vi "Set Handle on Open.vi"(0 "error in":errorcluster, 1 "All Handles ref":refnum<vi>, 2 "hDevice":i32, 3 "Selected Device":i32, 4 "Ch refs":refnum<vi>[](array[refnum]), 5 "OphirLMMeasurementLib.ICoLMMeasurement":refnum<k7>, 8 "Devices List box ref":refnum<vi>) -> ()   [LabVIEW 2017, in "Powermeter_library.lvlib"]
uses:
  Powermeter_library.lvlib
  Channel States.ctl
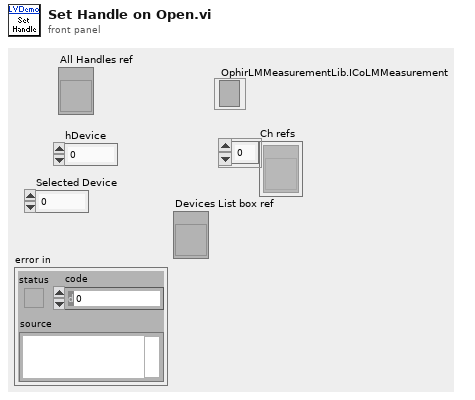
[diagram p1: front panel]
types:
  T1 = typedef "Powermeter_library.lvlib/Channel States.ctl" = enum16{"Init", "Poll", "Set Handle", "Measure"}
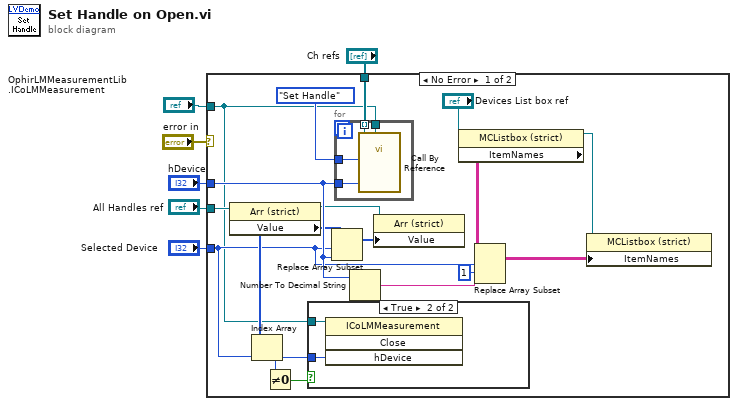
[diagram p0: block diagram]
diagram:
  n1 = case shown="No Error" "error in" {
    tunnel: "Selected Device" -> [w10 _]
    tunnel: "hDevice" -> [w19 _]
    tunnel: "Ch refs" -> [w21 _]
    tunnel: "OphirLMMeasurementLib.ICoLMMeasurement" -> [w7 _]
    tunnel: "All Handles ref" -> [w17 _]
    frame No Error {
      n2 = property class="Arr (strict)"(reference=w17) -> (reference out=w16:refnum<vi>, "Value"=w11:i32[])  [unwired: 1 in, 1 out]
      n3 = Index Array(array=w11, index=w10) -> (element=w8:i32)
      n4 = Not Equal To 0?(x=w8) -> (x != 0?=w9:bool)
      n5 = case shown="True" w9 {
        tunnel: w8 -> [_ w25]
        tunnel: w7 -> [_ w24]
        frame False {
        }
        frame True {
          n6 = invoke class="ICoLMMeasurement" method="Close"(reference=w24, "hDevice"=w25) -> ()  [unwired: 2 in, 4 out]
        }
      }
      n7 = Replace Array Subset(array=w11, new element=w19, index=w10) -> (w23:i32[])
      n8 = for {
        tunnel: w19 -> [w29]
        tunnel: Channel_States."Set Handle" ("State") -> [w28]
        tunnel: w21 -> [w27] mode=indexing
        tunnel: w7 -> [w26]
        n9 = call-by-ref "?"(reference=w27, "OphirLMMeasurementLib.ICoLMMeasurement"=w26, "Handle in"=w29, "State"=w28) -> ()  [unwired: 8 in, 3 out]
      }
      n10 = Number To Decimal String(number=w19) -> (decimal integer string=w18:string)  [unwired: 1 out]
      n11 = property class="Arr (strict)"(reference=w16, "Value"=w23) -> ()  [unwired: 1 in, 2 out]
      n12 = property class="MCListbox (strict)"(reference="Devices List box ref") -> (reference out=w13:refnum<vi>, "ItemNames"=w14:string[][])  [unwired: 1 in, 1 out]
      n13 = Replace Array Subset(array=w14, new element=w18, index (row)=w10, index (col)=1 ("disabled index (col)")) -> (w12:string[][])
      n14 = property class="MCListbox (strict)"(reference=w13, "ItemNames"=w12) -> ()  [unwired: 1 in, 2 out]
    }
    frame Error {
    }
  }
